vi "Purge with argon.vi"(9 "Prime pumps":bool, 10 "Control parameter":T1={"Pressure (psi)"=15.0, "Repeat times"=0, "Delayed time for waiting(s)"=0.0, "Refill rate\n(ml/min)"=6.0, "Refill volume (mL)"=1.0, "Infuse rate\n(ml/min)"=5.0, "Infuse volume (mL)"=1.0, "Sample loop prime volume (mL) "=1.0} {"Sample loop prime volume (mL)" format="%#.4f"; "Infuse volume (mL)" format="%#.4f"; "Infuse rate\n(ml/min)" format="%#.4f"; "Refill volume (mL)" format="%#.4f"; "Refill rate\n(ml/min)" format="%#.4f"}, 11 "Configured COM ports":T2={"Pump 1 COM"="COM12", "Pump 2 COM"="COM9", "Pump 3 COM"="COM13", "Pump 4 COM"="COM4", "Pump 5 COM"="COM4"}) -> ()   [LabVIEW 2017]
uses:
  <instrlib>/Harvard Apparatus PHD Ultra Series/Harvard Apparatus PHD Ultra Series.lvlib
  <instrlib>/Harvard Syringe Pump PHD2000/Harvard Syringe Pump PHD2000.lvlib
panel:
  out "Pump 5 COM":refnum<visa-resource-name>="COM12"
  out "Sample loop prime volume (mL)":dbl=1.0 format="%#.4f"
  out "Infuse volume (mL)":dbl=1.0 format="%#.4f"
  out "Infuse rate (ml/min)":dbl=5.0 format="%#.4f"
  out "Counter":i32
  out "Action selector":enum16{"Refill", "Infuse"}(ring)
  out "Repeat times":i32
  out "Delayed time for waiting(s)":dbl
  out "Refill volume (mL)":dbl=1.0 format="%#.4f"
  out "Refill rate (ml/min)":dbl=6.0 format="%#.4f"
  out "Pressure (psi)":dbl=15.0
  out "Pump 4 COM":refnum<visa-resource-name>="COM12"
  out "Pump 3 COM":refnum<visa-resource-name>="COM12"
  out "Pump 2 COM":refnum<visa-resource-name>="COM12"
  out "Pump 1 COM":refnum<visa-resource-name>="COM12"
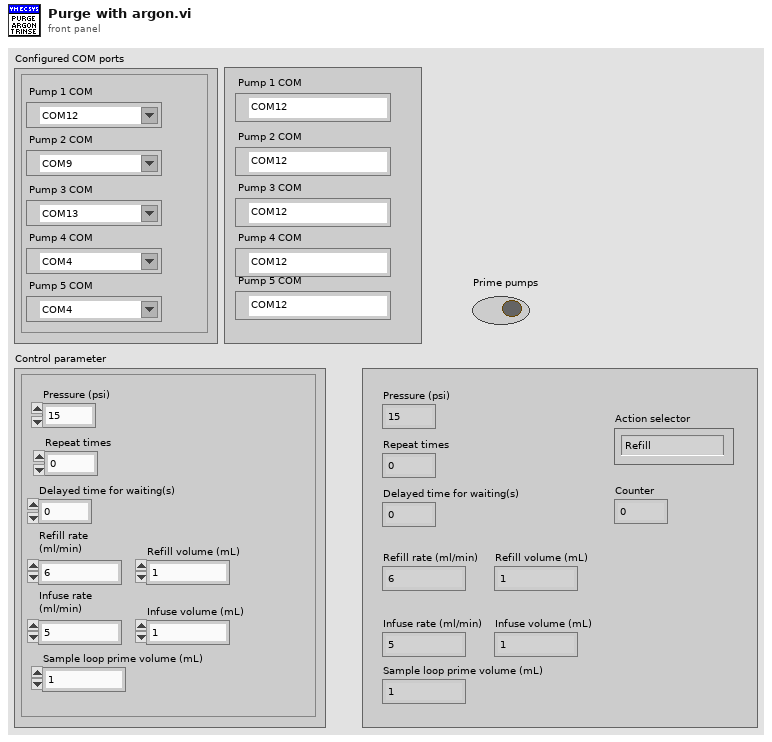
[diagram p1: front panel]
types:
  T1 = cluster{"Pressure (psi)":dbl, "Repeat times":i32, "Delayed time for waiting(s)":dbl, "Refill rate\n(ml/min)":dbl, "Refill volume (mL)":dbl, "Infuse rate\n(ml/min)":dbl, "Infuse volume (mL)":dbl, "Sample loop prime volume (mL) ":dbl}
  T2 = cluster{"Pump 1 COM":refnum<visa-resource-name>, "Pump 2 COM":refnum<visa-resource-name>, "Pump 3 COM":refnum<visa-resource-name>, "Pump 4 COM":refnum<visa-resource-name>, "Pump 5 COM":refnum<visa-resource-name>}
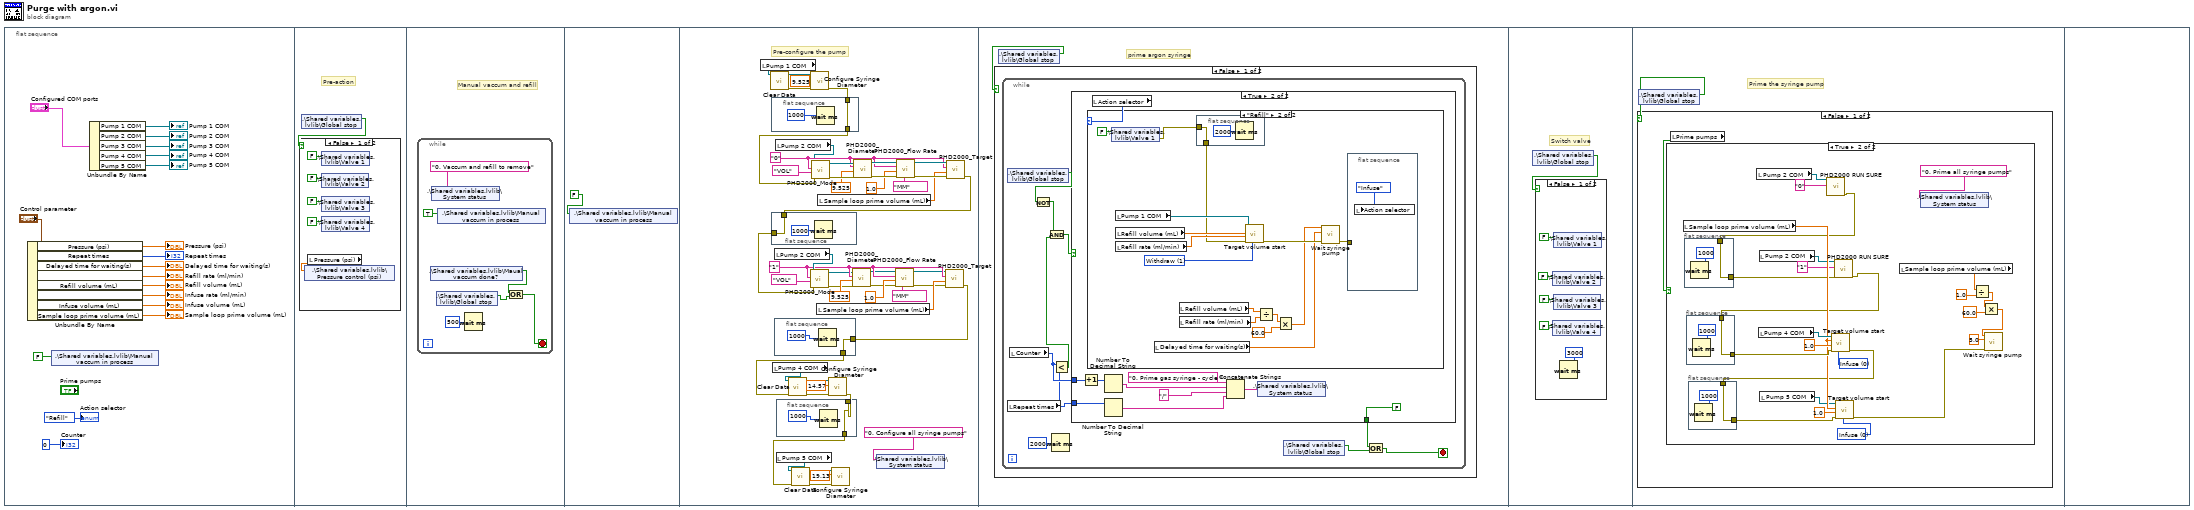
[diagram p0: block diagram]
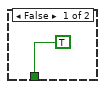
[diagram p3: hidden frame]
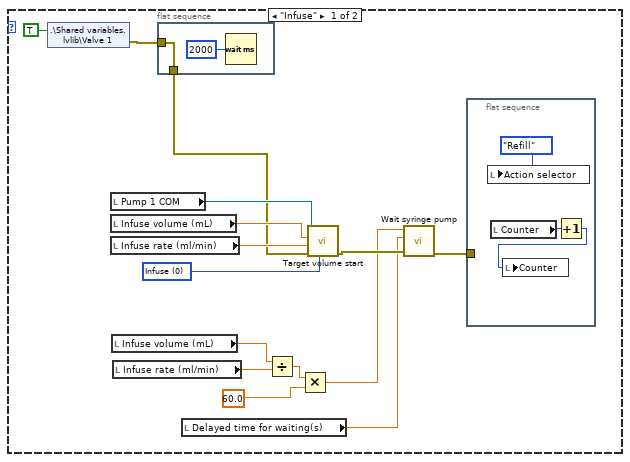
[diagram p4: hidden frame]
diagram:
  n1 = flat-sequence {
    frame #0 {
      n2 = Unbundle By Name("Control parameter") -> ("Pressure (psi)"=→"Pressure (psi)":dbl, "Repeat times"=→"Repeat times":i32, "Delayed time for waiting(s)"=→"Delayed time for waiting(s)":dbl, "Refill rate\n(ml/min)"=→"Refill rate (ml/min)":dbl, "Refill volume (mL)"=→"Refill volume (mL)":dbl, "Infuse rate\n(ml/min)"=→"Infuse rate (ml/min)":dbl, "Infuse volume (mL)"=→"Infuse volume (mL)":dbl, "Sample loop prime volume (mL)"=→"Sample loop prime volume (mL)":dbl)
      n3 = shared-variable ".\\Shared variables.lvlib\\Manual vaccum in process"(FALSE ("Manual vaccum in process")) -> ()  [unwired: 1 in, 1 out]
      n4 = Unbundle By Name("Configured COM ports") -> ("Pump 1 COM"=→"Pump 1 COM":refnum<visa-resource-name>, "Pump 2 COM"=→"Pump 2 COM":refnum<visa-resource-name>, "Pump 3 COM"=→"Pump 3 COM":refnum<visa-resource-name>, "Pump 4 COM"=→"Pump 4 COM":refnum<visa-resource-name>, "Pump 5 COM"=→"Pump 5 COM":refnum<visa-resource-name>)
      "Action selector" <- enum16{"Refill", "Infuse"}."Refill" ("Action selector")
      "Counter" <- 0 ("Counter")
    }
    frame #1 {
      # "Pre-action"
      n5 = shared-variable ".\\Shared variables.lvlib\\Global stop"() -> (w19:bool)  [unwired: 1 in, 1 out]
      n6 = case shown="False" w19 {
        frame False {
          n7 = local read "Pressure (psi)"() -> (w21:dbl)
          n8 = shared-variable ".\\Shared variables.lvlib\\Pressure control (psi)"(w21) -> ()  [unwired: 1 in, 1 out]
          n9 = shared-variable ".\\Shared variables.lvlib\\Valve 2"(FALSE ("Valve 2")) -> ()  [unwired: 1 in, 1 out]
          n10 = shared-variable ".\\Shared variables.lvlib\\Valve 1"(FALSE ("Valve 1")) -> ()  [unwired: 1 in, 1 out]
          n11 = shared-variable ".\\Shared variables.lvlib\\Valve 3"(FALSE ("Valve 3")) -> ()  [unwired: 1 in, 1 out]
          n12 = shared-variable ".\\Shared variables.lvlib\\Valve 4"(FALSE ("Valve 3")) -> ()  [unwired: 1 in, 1 out]
        }
        frame True {
        }
      }
    }
    frame #2 {
      # "Manual vaccum and refill"
      n13 = while {
        stop <- w27 stop-if-true
        n14 = shared-variable ".\\Shared variables.lvlib\\Maual vaccum done?"() -> (w29:bool)  [unwired: 1 in, 1 out]
        n15 = shared-variable ".\\Shared variables.lvlib\\System status"("0. Vaccum and refill to remove" ("System status")) -> ()  [unwired: 1 in, 1 out]
        n16 = shared-variable ".\\Shared variables.lvlib\\Global stop"() -> (w28:bool)  [unwired: 1 in, 1 out]
        n17 = shared-variable ".\\Shared variables.lvlib\\Manual vaccum in process"(TRUE ("Manual vaccum in process")) -> ()  [unwired: 1 in, 1 out]
        n18 = Wait (ms)(milliseconds to wait=u32 500) -> ()  [unwired: 1 out]
        n19 = Or(x=w29, y=w28) -> (x .or. y?=w27:bool)
      }
    }
    frame #3 {
      n20 = shared-variable ".\\Shared variables.lvlib\\Manual vaccum in process"(FALSE ("Manual vaccum in process")) -> ()  [unwired: 1 in, 1 out]
    }
    frame #4 {
      w44 = "1" ("Pump #")
      w52 = "0" ("Pump #")
      # "Pre-configure the pump"
      n21 = local read "Pump 1 COM"() -> (w76:refnum<visa-resource-name>)
      n22 = call <instrlib>:"Clear Data.vi"("VISA resource name"=w76) -> ("error out"=w78:errorcluster, "VISA resource name out"=w77:refnum<visa-resource-name>)  [unwired: 9 in]
      n23 = flat-sequence {
        tunnel: [w83] -> w34
        tunnel: w49 -> [w83]
        frame #0 {
          n24 = Wait (ms)(milliseconds to wait=u32 1000) -> ()  [unwired: 1 out]
        }
      }
      n25 = flat-sequence {
        tunnel: [w86] -> w54
        tunnel: w70 -> [w86]
        frame #0 {
          n26 = Wait (ms)(milliseconds to wait=u32 1000) -> ()  [unwired: 1 out]
        }
      }
      n27 = local read "Pump 4 COM"() -> (w71:refnum<visa-resource-name>)
      n28 = local read "Pump 2 COM"() -> (w46:refnum<visa-resource-name>)
      n29 = flat-sequence {
        tunnel: [w82] -> w69
        tunnel: w33 -> [w82]
        frame #0 {
          n30 = Wait (ms)(milliseconds to wait=u32 1000) -> ()  [unwired: 1 out]
        }
      }
      n31 = local read "Pump 2 COM"() -> (w50:refnum<visa-resource-name>)
      n32 = flat-sequence {
        tunnel: [w80] -> w63
        tunnel: w68 -> [w80]
        frame #0 {
          n33 = Wait (ms)(milliseconds to wait=u32 1000) -> ()  [unwired: 1 out]
        }
      }
      n34 = local read "Pump 5 COM"() -> (w67:refnum<visa-resource-name>)
      n35 = call <instrlib>:"Clear Data.vi"("error in (no error)"=w69, "VISA resource name"=w71) -> ("error out"=w74:errorcluster, "VISA resource name out"=w73:refnum<visa-resource-name>)  [unwired: 8 in]
      n36 = call <instrlib>:"Clear Data.vi"("error in (no error)"=w63, "VISA resource name"=w67) -> ("error out"=w64:errorcluster, "VISA resource name out"=w65:refnum<visa-resource-name>)  [unwired: 8 in]
      n37 = call <instrlib>:"PHD2000_Mode.vi"("error in (no error)"=w34, "Mode"="VOL", "Pump #"=w44, "VISA resource name 2"=w46) -> ("error out"=w41:errorcluster, "VISA resource name out"=w40:refnum<visa-resource-name>)  [unwired: 5 in, 1 out]
      n38 = call <instrlib>:"Configure Syringe Diameter.vi"("error in (no error)"=w78, "Syringe Diameter (20 mm)"=9.525, "VISA resource name"=w77) -> ("error out"=w70:errorcluster)  [unwired: 7 in, 1 out]
      n39 = call <instrlib>:"PHD2000_Mode.vi"("error in (no error)"=w54, "Mode"="VOL", "Pump #"=w52, "VISA resource name 2"=w50) -> ("error out"=w56:errorcluster, "VISA resource name out"=w57:refnum<visa-resource-name>)  [unwired: 5 in, 1 out]
      n40 = local read "Sample loop prime volume (mL)"() -> (w47:dbl)
      n41 = local read "Sample loop prime volume (mL)"() -> (w48:dbl)
      n42 = call <instrlib>:"Configure Syringe Diameter.vi"("error in (no error)"=w74, "Syringe Diameter (20 mm)"=14.57, "VISA resource name"=w73) -> ("error out"=w68:errorcluster)  [unwired: 7 in, 1 out]
      n43 = call <instrlib>:"Configure Syringe Diameter.vi"("error in (no error)"=w64, "Syringe Diameter (20 mm)"=19.13, "VISA resource name"=w65) -> ()  [unwired: 7 in, 2 out]
      n44 = call <instrlib>:"PHD2000_Diameter.vi"("VISA resource name 2"=w40, "Pump #"=w44, "diameter (mm)"=9.525 ("Syringe Diameter (20 mm)"), "error in (no error)"=w41) -> ("VISA resource name out"=w38:refnum<visa-resource-name>, "error out"=w36:errorcluster)  [unwired: 5 in]
      n45 = call <instrlib>:"PHD2000_Diameter.vi"("VISA resource name 2"=w57, "Pump #"=w52, "diameter (mm)"=9.525 ("Syringe Diameter (20 mm)"), "error in (no error)"=w56) -> ("VISA resource name out"=w59:refnum<visa-resource-name>, "error out"=w61:errorcluster)  [unwired: 5 in]
      n46 = shared-variable ".\\Shared variables.lvlib\\System status"("0. Configure all syringe pumps" ("System status")) -> ()  [unwired: 1 in, 1 out]
      n47 = call <instrlib>:"PHD2000_Flow Rate.vi"("VISA resource name 2"=w38, "Pump #"=w44, "flowrate"=1.0, "error in (no error)"=w36, "Unit"="MM") -> ("VISA resource name out"=w37:refnum<visa-resource-name>, "error out"=w35:errorcluster)  [unwired: 4 in]
      n48 = call <instrlib>:"PHD2000_Flow Rate.vi"("VISA resource name 2"=w59, "Pump #"=w52, "flowrate"=1.0, "error in (no error)"=w61, "Unit"="MM") -> ("VISA resource name out"=w60:refnum<visa-resource-name>, "error out"=w62:errorcluster)  [unwired: 4 in]
      n49 = call <instrlib>:"PHD2000_Target.vi"("error in (no error)"=w35, "Target (ml)"=w47, "Pump #"=w44, "VISA resource name 2"=w37) -> ("error out"=w33:errorcluster)  [unwired: 5 in, 2 out]
      n50 = call <instrlib>:"PHD2000_Target.vi"("error in (no error)"=w62, "Target (ml)"=w48, "Pump #"=w52, "VISA resource name 2"=w60) -> ("error out"=w49:errorcluster)  [unwired: 5 in, 2 out]
    }
    frame #5 {
      # "prime argon syringe"
      n51 = shared-variable ".\\Shared variables.lvlib\\Global stop"() -> (w87:bool)  [unwired: 1 in, 1 out]
      n52 = case shown="False" w87 {
        frame False {
          n53 = while {
            stop <- w97 stop-if-true
            n54 = shared-variable ".\\Shared variables.lvlib\\Global stop"() -> (w93:bool)  [unwired: 1 in, 1 out]
            n55 = local read "Repeat times"() -> (w88:i32)
            n56 = local read "Counter"() -> (w89:i32)
            n57 = Not(x=w93) -> (.not. x?=w92:bool)
            n58 = Wait (ms)(milliseconds to wait=u32 2000) -> ()  [unwired: 1 out]
            n59 = Less?(x=w89, y=w88) -> (x < y?=w91:bool)
            n60 = And(x=w92, y=w91) -> (x .and. y?=w90:bool)
            n61 = case shown="True" w90 {
              tunnel: [TRUE FALSE] -> w96
              tunnel: w89 -> [_ w102]
              tunnel: w88 -> [_ w100]
              frame False {
              }
              frame True {
                n62 = Increment(x=w102) -> (x+1=w101:i32)
                n63 = local read "Action selector"() -> (w108:enum16{"Refill", "Infuse"})
                n64 = case shown="\"Refill\"" w108 {
                  frame "Infuse" {
                    w117 = u16 0 items=["Infuse", "Withdraw"] ("Pump Direction (0:Infuse)")
                    n65 = shared-variable ".\\Shared variables.lvlib\\Valve 1"(TRUE ("Valve 1")) -> (error out=w118:errorcluster)  [unwired: 1 in]
                    n66 = local read "Pump 1 COM"() -> (w114:refnum<visa-resource-name>)
                    n67 = local read "Infuse volume (mL)"() -> (w115:dbl)
                    n68 = local read "Infuse rate (ml/min)"() -> (w116:dbl)
                    n69 = local read "Infuse volume (mL)"() -> (w120:dbl)
                    n70 = local read "Infuse rate (ml/min)"() -> (w121:dbl)
                    n71 = flat-sequence {
                      tunnel: [w124] -> w113
                      tunnel: w118 -> [w124]
                      frame #0 {
                        n72 = Wait (ms)(milliseconds to wait=u32 2000) -> ()  [unwired: 1 out]
                      }
                    }
                    n73 = local read "Delayed time for waiting(s)"() -> (w109:dbl)
                    n74 = Divide(x=w120, y=w121) -> (x/y=w123:dbl)
                    n75 = Multiply(x=w123, y=60.0) -> (x*y=w110:dbl)
                    n76 = call "Target volume start.vi"("Pump Direction (0:Infuse)"=w117, "error in (no error)"=w113, "Flow Rate (ml/min)"=w116, "Target volume (ml)"=w115, "VISA resource name"=w114) -> ("error out"=w112:errorcluster)  [unwired: 5 in, 1 out]
                    n77 = call "Wait syringe pump.vi"("error in (no error)"=w112, "Delayed time (s)"=w109, "Time Target (s)"=w110) -> ("error out"=w111:errorcluster)  [unwired: 8 in]
                    n78 = flat-sequence {
                      tunnel: w111 -> [_]
                      frame #0 {
                        n79 = local write "Action selector"(enum16{"Refill", "Infuse"}."Refill" ("Action selector")) -> ()
                        n80 = local read "Counter"() -> (w127:i32)
                        n81 = Increment(x=w127) -> (x+1=w126:i32)
                        n82 = local write "Counter"(w126) -> ()
                      }
                    }
                  }
                  frame "Refill" {
                    w137 = u16 1 items=["Infuse", "Withdraw"] ("Pump Direction (0:Infuse)")
                    n83 = shared-variable ".\\Shared variables.lvlib\\Valve 1"(FALSE ("Valve 1")) -> (error out=w138:errorcluster)  [unwired: 1 in]
                    n84 = local read "Pump 1 COM"() -> (w134:refnum<visa-resource-name>)
                    n85 = local read "Refill volume (mL)"() -> (w135:dbl)
                    n86 = local read "Refill rate (ml/min)"() -> (w136:dbl)
                    n87 = local read "Delayed time for waiting(s)"() -> (w129:dbl)
                    n88 = local read "Refill volume (mL)"() -> (w142:dbl)
                    n89 = local read "Refill rate (ml/min)"() -> (w141:dbl)
                    n90 = flat-sequence {
                      tunnel: [w144] -> w133
                      tunnel: w138 -> [w144]
                      frame #0 {
                        n91 = Wait (ms)(milliseconds to wait=u32 2000) -> ()  [unwired: 1 out]
                      }
                    }
                    n92 = call "Target volume start.vi"("Pump Direction (0:Infuse)"=w137, "error in (no error)"=w133, "Flow Rate (ml/min)"=w136, "Target volume (ml)"=w135, "VISA resource name"=w134) -> ("error out"=w132:errorcluster)  [unwired: 5 in, 1 out]
                    n93 = Divide(x=w142, y=w141) -> (x/y=w143:dbl)
                    n94 = Multiply(x=w143, y=60.0) -> (x*y=w130:dbl)
                    n95 = call "Wait syringe pump.vi"("error in (no error)"=w132, "Delayed time (s)"=w129, "Time Target (s)"=w130) -> ("error out"=w131:errorcluster)  [unwired: 8 in]
                    n96 = flat-sequence {
                      tunnel: w131 -> [_]
                      frame #0 {
                        n97 = local write "Action selector"(enum16{"Refill", "Infuse"}."Infuse" ("Action selector")) -> ()
                      }
                    }
                  }
                }
                n98 = Number To Decimal String(number=w101) -> (decimal integer string=w105:string)  [unwired: 1 in]
                n99 = Number To Decimal String(number=w100) -> (decimal integer string=w99:string)  [unwired: 1 in]
                n100 = Concatenate Strings("0. Prime gas syringe - cycle " ("System status"), w105, "/" ("string"), w99) -> (w104:string)
                n101 = shared-variable ".\\Shared variables.lvlib\\System status"(w104) -> ()  [unwired: 1 in, 1 out]
              }
            }
            n102 = shared-variable ".\\Shared variables.lvlib\\Global stop"() -> (w95:bool)  [unwired: 1 in, 1 out]
            n103 = Or(x=w96, y=w95) -> (x .or. y?=w97:bool)
          }
        }
        frame True {
        }
      }
    }
    frame #6 {
      # "Switch valve"
      n104 = shared-variable ".\\Shared variables.lvlib\\Global stop"() -> (w147:bool)  [unwired: 1 in, 1 out]
      n105 = case shown="False" w147 {
        frame False {
          n106 = shared-variable ".\\Shared variables.lvlib\\Valve 2"(FALSE ("Valve 2")) -> ()  [unwired: 1 in, 1 out]
          n107 = shared-variable ".\\Shared variables.lvlib\\Valve 4"(FALSE ("Valve 3")) -> ()  [unwired: 1 in, 1 out]
          n108 = shared-variable ".\\Shared variables.lvlib\\Valve 3"(FALSE ("Valve 3")) -> ()  [unwired: 1 in, 1 out]
          n109 = shared-variable ".\\Shared variables.lvlib\\Valve 1"(FALSE ("Valve 1")) -> ()  [unwired: 1 in, 1 out]
          n110 = Wait (ms)(milliseconds to wait=u32 3000) -> ()  [unwired: 1 out]
        }
        frame True {
        }
      }
    }
    frame #7 {
      # "Prime the syringe pump"
      n111 = shared-variable ".\\Shared variables.lvlib\\Global stop"() -> (w153:bool)  [unwired: 1 in, 1 out]
      n112 = case shown="False" w153 {
        frame False {
          n113 = local read "Prime pumps"() -> (w154:bool)
          n114 = case shown="True" w154 {
            frame False {
            }
            frame True {
              w168 = u16 0 items=["Infuse", "Withdraw"] ("Pump Direction (0:Infuse)")
              w178 = u16 0 items=["Infuse", "Withdraw"] ("Pump Direction (0:Infuse)")
              n115 = local read "Sample loop prime volume (mL)"() -> (w169:dbl)
              n116 = flat-sequence {
                tunnel: w160 -> [w180]
                tunnel: [w180] -> w158
                frame #0 {
                  n117 = Wait (ms)(milliseconds to wait=u32 1000) -> ()  [unwired: 1 out]
                }
              }
              n118 = flat-sequence {
                tunnel: w159 -> [w184]
                tunnel: [w184] -> w176
                frame #0 {
                  n119 = Wait (ms)(milliseconds to wait=u32 1000) -> ()  [unwired: 1 out]
                }
              }
              n120 = flat-sequence {
                tunnel: w167 -> [w182]
                tunnel: [w182] -> w166
                frame #0 {
                  n121 = Wait (ms)(milliseconds to wait=u32 1000) -> ()  [unwired: 1 out]
                }
              }
              n122 = local read "Pump 2 COM"() -> (w161:refnum<visa-resource-name>)
              n123 = local read "Pump 4 COM"() -> (w179:refnum<visa-resource-name>)
              n124 = local read "Pump 2 COM"() -> (w156:refnum<visa-resource-name>)
              n125 = local read "Pump 5 COM"() -> (w164:refnum<visa-resource-name>)
              n126 = call "PHD2000 RUN SURE.vi"("Pump #"="0", "VISA resource name 2"=w161) -> ("error out"=w160:errorcluster)  [unwired: 8 in, 1 out]
              n127 = call "Target volume start.vi"("Pump Direction (0:Infuse)"=w178, "error in (no error)"=w176, "Flow Rate (ml/min)"=1.0 ("Flow Rate (5.00)"), "Target volume (ml)"=w169, "VISA resource name"=w179) -> ("error out"=w167:errorcluster)  [unwired: 5 in, 1 out]
              n128 = call "PHD2000 RUN SURE.vi"("error in (no error)"=w158, "Pump #"="1", "VISA resource name 2"=w156) -> ("error out"=w159:errorcluster)  [unwired: 7 in, 1 out]
              n129 = call "Target volume start.vi"("Pump Direction (0:Infuse)"=w168, "error in (no error)"=w166, "Flow Rate (ml/min)"=1.0, "Target volume (ml)"=w169, "VISA resource name"=w164) -> ("error out"=w163:errorcluster)  [unwired: 5 in, 1 out]
              n130 = local read "Sample loop prime volume (mL)"() -> (w174:dbl)
              n131 = shared-variable ".\\Shared variables.lvlib\\System status"("0. Prime all syringe pumps" ("System status")) -> ()  [unwired: 1 in, 1 out]
              n132 = Divide(x=w174, y=1.0) -> (x/y=w175:dbl)
              n133 = Multiply(x=w175, y=60.0) -> (x*y=w171:dbl)
              n134 = call "Wait syringe pump.vi"("error in (no error)"=w163, "Delayed time (s)"=5.0, "Time Target (s)"=w171) -> ()  [unwired: 8 in, 1 out]
            }
          }
        }
        frame True {
        }
      }
    }
    frame #8 {
    }
  }
